vi "RANGE Zero Error Offset.vi"(8 "Error In":errorcluster, 10 "FMA1600A Gas Data in":T1, 11 "SLPM Error @ Zero":dbl) -> (0 "Error Out":errorcluster, 3 "FMA1600A Gas Data out":T1)   [LabVIEW 2018]
uses:
  Drivers/Omega FMA-1600A Series Gas Flow Meter/Type Definitions/FMA1600A Data.ctl
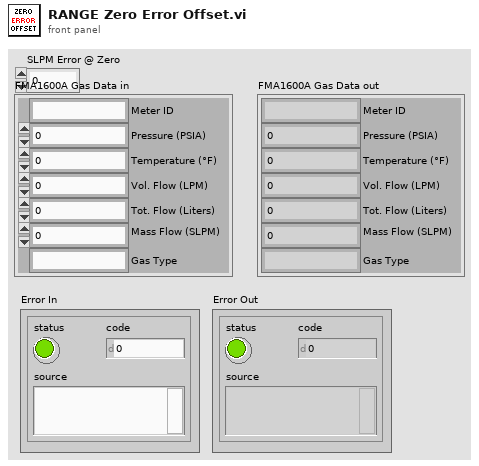
[diagram p1: front panel]
types:
  T1 = typedef "FMA1600A Data.ctl" = cluster{"Pressure (PSIA)":dbl, "Temperature (°F)":dbl, "Vol. Flow (LPM)":dbl, "Mass Flow (SLPM)":dbl, "Gas Type":string, "Tot. Flow (Liters)":dbl, "Meter ID":string}
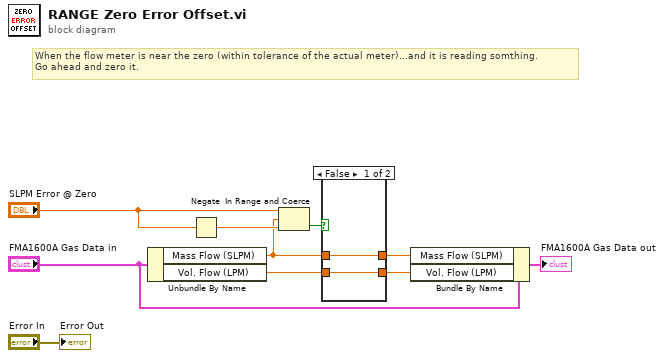
[diagram p0: block diagram]
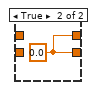
[diagram p2: hidden frame]
diagram:
  # "When the flow meter is near the zero (within tolerance of the actual meter)...and it is reading somthing.\nGo ahead and zero it."
  n1 = Unbundle By Name("FMA1600A Gas Data in") -> ("Mass Flow (SLPM)"=w2:dbl, "Vol. Flow (LPM)"=w1:dbl)
  n2 = Negate(x="SLPM Error @ Zero") -> (-x=w6:dbl)
  n3 = In Range and Coerce(upper limit="SLPM Error @ Zero", x=w2, lower limit=w6) -> (In Range?=w5:bool)  [unwired: 1 out]
  n4 = case shown="False" w5 {
    tunnel: [w12 w13] -> w4
    tunnel: [w11 w13] -> w3
    tunnel: w2 -> [w12 _]
    tunnel: w1 -> [w11 _]
    frame False {
    }
    frame True {
      w13 = 0.0
    }
  }
  n5 = Bundle By Name(cluster="FMA1600A Gas Data in", "Mass Flow (SLPM)"=w4, "Vol. Flow (LPM)"=w3) -> (→"FMA1600A Gas Data out":T1)
  "Error Out" <- "Error In"
